vi "Apply move.vi"(8 "error in (no error)":errorcluster, 10 "Position in":refnum<class "Position.lvclass">, 11 "Move in":refnum<class "Move.lvclass">) -> (0 "error out":errorcluster, 2 "Position out":refnum<class "Position.lvclass">, 3 "Move out":refnum<class "Move.lvclass">)   [LabVIEW 2016, in "Chesslib.lvlib" / "Move.lvclass"]
uses:
  Move.lvclass
  Position/Position.lvclass
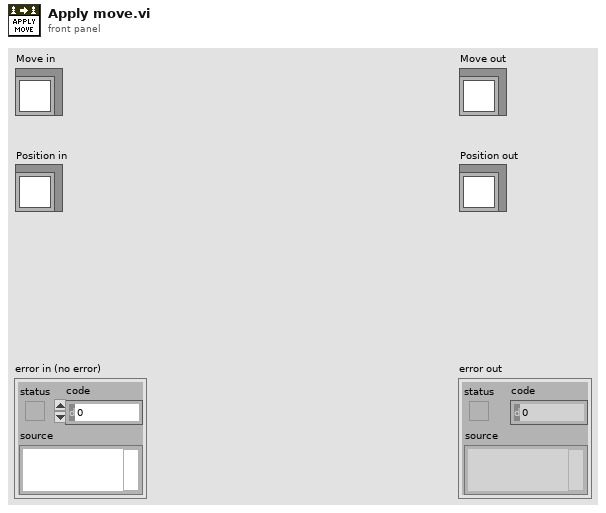
[diagram p1: front panel]
types:
  T1 = typedef "Chesslib.lvlib/Square.ctl" = cluster{"File":T2, "Rank":T3}
  T2 = typedef "Chesslib.lvlib/File.ctl" = enum8{"a", "b", "c", "d", "e", "f", "g", "h"}
  T3 = typedef "Chesslib.lvlib/Rank.ctl" = enum8{"1", "2", "3", "4", "5", "6", "7", "8"}
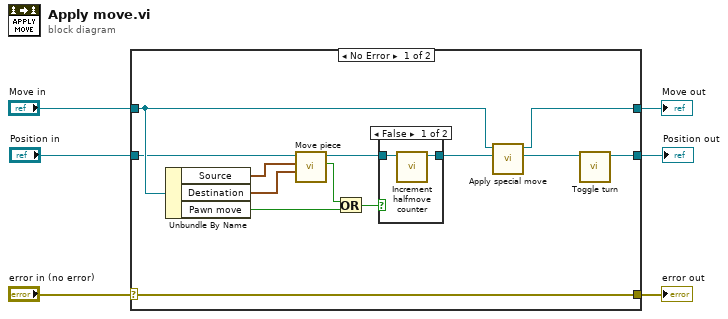
[diagram p0: block diagram]
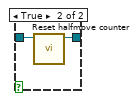
[diagram p2: hidden frame]
diagram:
  n1 = case shown="No Error" "error in (no error)" {
    selector: "error in (no error)" -> [w19 w26]
    tunnel: [w19 w26] -> w5
    tunnel: [w10 w25] -> w3
    tunnel: "Move in" -> [w15 w25]
    tunnel: [w17 w24] -> w2
    tunnel: "Position in" -> [w12 w24]
    frame No Error {
      n2 = Unbundle By Name(w15) -> ("Source"=w11:T1, "Destination"=w16:T1, "Pawn move"=w13:bool)
      n3 = call "Move piece.vi"("Destination"=w16, "Source"=w11, "Position in"=w12) -> ("Capture?"=w14:bool, "Position out"=w9:refnum<class "Position.lvclass">)  [unwired: 5 in, 2 out]
      n4 = Or(x=w14, y=w13) -> (x .or. y?=w18:bool)
      n5 = case shown="False" w18 {
        tunnel: w9 -> [w21 w23]
        tunnel: [w20 w22] -> w8
        frame False {
          n6 = call "Increment halfmove counter.vi"("Position in"=w21) -> ("Position out"=w20:refnum<class "Position.lvclass">)  [unwired: 9 in, 1 out]
        }
        frame True {
          n7 = call "Reset halfmove counter.vi"("Position in"=w23) -> ("Position out"=w22:refnum<class "Position.lvclass">)  [unwired: 9 in, 1 out]
        }
      }
      n8 = call-dynamic "Apply special move.vi"("Position in"=w8, "Move in"=w15) -> ("Position out"=w7:refnum<class "Position.lvclass">, "Move out"=w10:refnum<class "Move.lvclass">)  [unwired: 7 in, 1 out]
      n9 = call "Toggle turn.vi"("Position in"=w7) -> ("Position out"=w17:refnum<class "Position.lvclass">)  [unwired: 9 in, 1 out]
    }
    frame Error {
    }
  }
  "error out" <- w5
  "Move out" <- w3
  "Position out" <- w2
